vi "GradosCentigrados.vi"() -> ()   [LabVIEW 2018]
panel:
  in  "Selecciona Grados Iniciales":bool
  out "Conversion":dbl
  in  "Grado":dbl
  in  "stop":bool
  # "°C"
  # "°F"
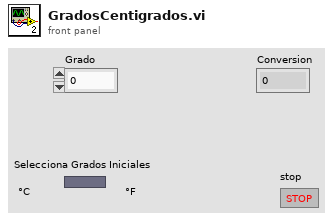
[diagram p1: front panel]
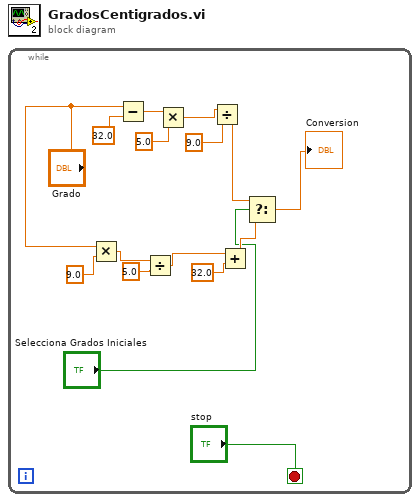
[diagram p0: block diagram]
diagram:
  n1 = while {
    stop <- "stop" stop-if-true
    n2 = Multiply(x="Grado", y=9.0) -> (x*y=w6:dbl)
    n3 = Subtract(x="Grado", y=32.0) -> (x-y=w12:dbl)
    n4 = Divide(x=w6, y=5.0) -> (x/y=w7:dbl)
    n5 = Multiply(x=w12, y=5.0) -> (x*y=w11:dbl)
    n6 = Divide(x=w11, y=9.0) -> (x/y=w4:dbl)
    n7 = Add(x=w7, y=32.0) -> (x+y=w5:dbl)
    n8 = Select(t=w4, s="Selecciona Grados Iniciales", f=w5) -> (s? t:f=→"Conversion":dbl)
  }
